vi "Do.vi"(8 "error in (no error)":errorcluster, 10 "Actor in":refnum<class "Actor.lvclass">, 11 "Get Result Msg":refnum<class "Get Result Msg.lvclass">) -> (0 "error out":errorcluster, 2 "Actor out":refnum<class "Actor.lvclass">)   [LabVIEW 2013, in "Calculate.lvlib" / "Get Result Msg.lvclass"]
doc: "This VI delivers the message to the actor by calling the appropriate method(s) on the actor."
uses:
  Get Result Msg.lvclass
  <vilib>/ActorFramework/Actor/Actor.lvclass
  Calculate/Calculate.lvclass
  Simulation/Simulation Data_Global.vi
  Simulation/Simulation.lvlib
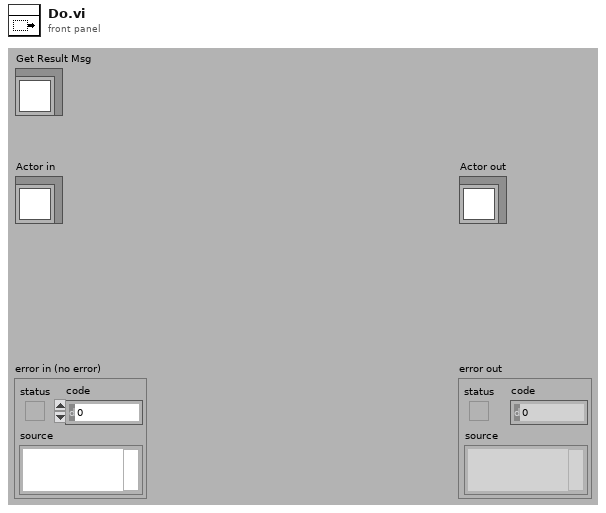
[diagram p1: front panel]
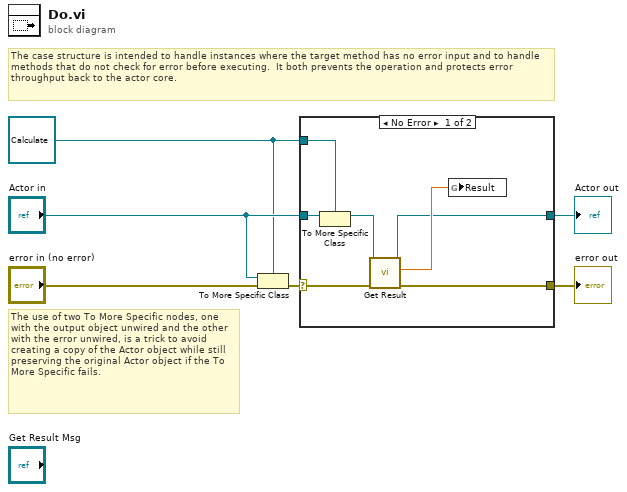
[diagram p0: block diagram]
diagram:
  w1 = refnum<class "Calculate.lvclass"> refnum ("Actor in")
  # "The use of two To More Specific nodes, one with the output object unwired and the other with the error unwired, is a trick to avoid creating a copy of the Actor object while still preserving the original Actor object if the To More Specific fails."
  # "The case structure is intended to handle instances where the target method has no error input and to handle methods that do not check for error before executing.  It both prevents the operation and protects error throughput back to the actor core."
  n1 = To More Specific Class(target class=w1, reference="Actor in", error in="error in (no error)") -> (error out=w5:errorcluster)  [unwired: 1 out]
  n2 = case shown="No Error" w5 {
    selector: w5 -> [w13 w15]
    tunnel: [w8 w15] -> w4
    tunnel: [w9 w14] -> w3
    tunnel: "Actor in" -> [w12 w14]
    tunnel: w1 -> [w7 _]
    frame No Error {
      n3 = To More Specific Class(target class=w7, reference=w12) -> (specific class reference=w11:refnum<class "Calculate.lvclass">)  [unwired: 1 in, 1 out]
      n4 = call-dynamic "Get Result.vi"("error in (no error)"=w13, "Calculate in"=w11) -> ("error out"=w8:errorcluster, "Result"=w10:dbl, "Calculate out"=w9:refnum<class "Calculate.lvclass">)  [unwired: 7 in]
      n5 = global write "Simulation Data_Global.vi" "Result"(w10) -> ()
    }
    frame Error {
      # "If type check fails, pass the original object out again."
    }
  }
  "error out" <- w4
  "Actor out" <- w3
